vi "002EH_DO_串口停止位写入.vi"(8 "error in (no error)":errorcluster caption="错误输入（无错误）", 10 "数值":enum16{"1bit", "2bit"}(ring), 11 "MB session in":refnum<class "MB_Master.lvclass">) -> (0 "error out":errorcluster caption="错误输出", 3 "MB session out":refnum<class "MB_Master.lvclass">)   [LabVIEW 2016, in "斯坦道多参数.lvlib"]
uses:
  <vilib>/Plasmionique/MB Master/MB Master.lvlib
  <vilib>/Plasmionique/MB Master/MB_Master/MB_Master.lvclass
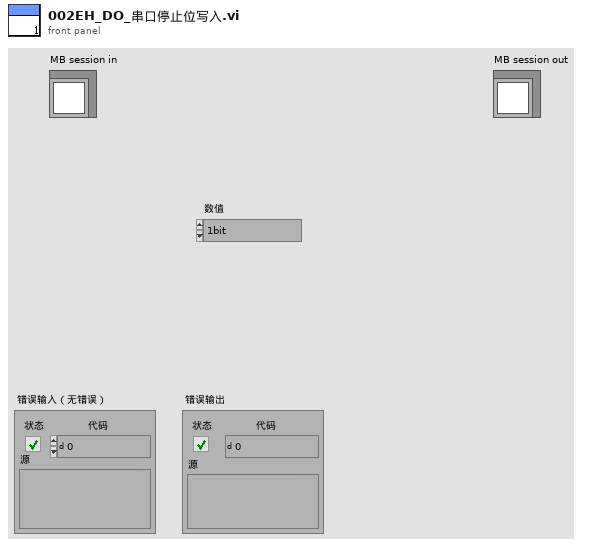
[diagram p1: front panel]
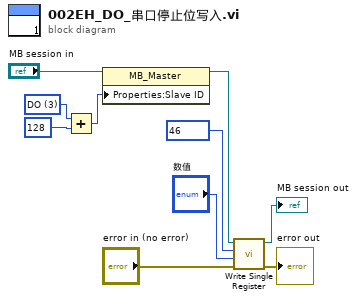
[diagram p0: block diagram]
diagram:
  w6 = u16 3 items=["NULL", "pH", "Cond", "DO", "Turb"] ("数值")
  n1 = Add(x=w6, y=u16 128) -> (x+y=w5:u16)
  n2 = property class="MB_Master"(reference="MB session in", "Properties:Slave ID"=w5) -> (reference out=w3:refnum<class "MB_Master.lvclass">)  [unwired: 1 in, 1 out]
  n3 = call <vilib>:"Write Single Register.vi"("error in (no error)"="error in (no error)", "value"="数值", "address"=u16 46 ("starting address"), "MB session in"=w3) -> ("error out"=→"error out":errorcluster, "MB session out"=→"MB session out":refnum<class "MB_Master.lvclass">)  [unwired: 6 in]
